vi "FindMinimumChiSquaredFastUncalibratedMethod.vi"(8 "Restrict to Positive Imaginary Part":bool=TRUE, 9 "Starting points 2":dbl[][](array[numeric])=[[1.5, 0.1], [1.5, 0.11], [1.52, 0.1]] format="%.6g", 10 "Simplex Graph":refnum<vi>, 11 "Extinction ExtinctionUncertainity Size parameter and Number ofS sizes":T1={"PAS amplitude"=[1.9915476e-09, 2.5260327e-09, 2.9463496e-09, 3.6659398e-09, 4.1150909e-09, 4.3561701e-09, 4.8158371e-09, 5.5805258e-09], "PAS amp Uncertainty"=[1.1685435e-10, 1.8562181e-10, 2.4682015e-10, 3.9807269e-10, 5.4913102e-10, 1.091901e-09, 1.2235488e-09, 1.7175431e-09], "Size parameters"=[2.4744035643168516, 2.699349342891111, 2.92429512146537, 3.149240900039629, 3.3741866786138885, 3.599132457188148, 3.8240782357624066, 4.049024014336666], "Number ofSizes"=8.0, "GeometricCrossSection"=[5.939573610693203e-10, 7.068583470577035e-10, 8.295768100885549e-10, 9.621127501618742e-10, 1.1044661672776617e-09, 1.2566370614359174e-09, 1.418625432636641e-09, 1.590431280879833e-09], "Wave Length"=349.14999, "SMPS Sizes"=[105.5, 109.4, 113.4, 117.6, 121.9, 126.3, 131.0, 135.8, 140.7, 145.9, 151.2, 156.8, 162.5, 168.5, 174.7, 181.1, 187.7, 194.6, 201.7, 209.1, 216.7, 224.7, 232.9, 241.4, 250.3, 259.5, 269.0, 278.8, 289.0, 299.6, 310.6, 322.0, 333.8, 346.0, 358.7, 371.8, 385.4, 399.5, 414.2, 429.4, 445.1, 461.4, 478.3, 495.8, 514.0, 532.8, 552.3, 572.5, 593.5, 615.3, 637.8, 661.2, 685.4, 710.5, 736.5, 763.5, 791.5], "Concentration"=array8x57[456 elements], "Double Charge Correction"=TRUE, "Extincation Factor"=1.0, "Diameter Factor"=1.0, "Diameter Offset"=0.0, "Extinction Factor Flag"=FALSE, "Diameter Factor Flag"=FALSE, "Diameter Offset Flag"=FALSE, "Sizes"=[275.0, 300.0, 325.0, 350.0, 375.0, 400.0, 425.0, 450.0], "ExtinctionOrAbsorptionOrScattering"=0, "Concentration(#/cc)"=[]} {"ExtinctionOrAbsorptionOrScattering" scale=0.0..2.0}) -> (1 "Imaginary Part from fit":dbl=0.051495699826118665, 2 "Real Part from fit":dbl=1.57799797397569, 3 "Extinction ExtinctionUncertainity Size parameter and Number ofS sizes 2":T1={"PAS amplitude"=[1.9915476e-09, 2.5260327e-09, 2.9463496e-09, 3.6659398e-09, 4.1150909e-09, 4.3561701e-09, 4.8158371e-09, 5.5805258e-09], "PAS amp Uncertainty"=[1.1685435e-10, 1.8562181e-10, 2.4682015e-10, 3.9807269e-10, 5.4913102e-10, 1.091901e-09, 1.2235488e-09, 1.7175431e-09], "Size parameters"=[2.4744035643168516, 2.699349342891111, 2.92429512146537, 3.149240900039629, 3.3741866786138885, 3.599132457188148, 3.8240782357624066, 4.049024014336666], "Number ofSizes"=8.0, "GeometricCrossSection"=[5.939573610693203e-10, 7.068583470577035e-10, 8.295768100885549e-10, 9.621127501618742e-10, 1.1044661672776617e-09, 1.2566370614359174e-09, 1.418625432636641e-09, 1.590431280879833e-09], "Wave Length"=349.14999, "SMPS Sizes"=[105.5, 109.4, 113.4, 117.6, 121.9, 126.3, 131.0, 135.8, 140.7, 145.9, 151.2, 156.8, 162.5, 168.5, 174.7, 181.1, 187.7, 194.6, 201.7, 209.1, 216.7, 224.7, 232.9, 241.4, 250.3, 259.5, 269.0, 278.8, 289.0, 299.6, 310.6, 322.0, 333.8, 346.0, 358.7, 371.8, 385.4, 399.5, 414.2, 429.4, 445.1, 461.4, 478.3, 495.8, 514.0, 532.8, 552.3, 572.5, 593.5, 615.3, 637.8, 661.2, 685.4, 710.5, 736.5, 763.5, 791.5], "Concentration"=array8x57[456 elements], "Double Charge Correction"=TRUE, "Extincation Factor"=1.0, "Diameter Factor"=1.0, "Diameter Offset"=0.0, "Extinction Factor Flag"=FALSE, "Diameter Factor Flag"=FALSE, "Diameter Offset Flag"=FALSE, "Sizes"=[275.0, 300.0, 325.0, 350.0, 375.0, 400.0, 425.0, 450.0], "ExtinctionOrAbsorptionOrScattering"=0, "Concentration(#/cc)"=[]} {"ExtinctionOrAbsorptionOrScattering" scale=0.0..2.0})   [LabVIEW 2013]
uses:
  BaesDataTypeDefinition.ctl
  RTDownhillSimplex.llb/RTDownhillSimplexGlobals.vi
panel:
  in  "Chi2 tolerance":dbl=0.001
  out "Waveform Chart":i32(graph)=60
  out "Starting points 3":dbl[][](array[numeric])=[[1.6630594557043747, 0.246532961950036], [1.4605000230939145, 0.15705446819563057], [1.5705619064033547, 0.05175990620612842]]
  in  "Downhill-Simplex parameters 2":T2={"alpha"=1.0, "beta"=0.5, "gamma"=2.0, "Maximum"=FALSE}
  out "Stopping condition flag":bool=TRUE
  out "x-y":dbl[](array[numeric])=[0.000168992022227199, 0.00018933075538369454]
  in  "buzzer":bool
  in  "Continous":bool=TRUE
  in  "sleep-time":dbl
  out "Simplex":cluster{dbl[], dbl[]}[](graph)=[{[1.57799797397569, 1.5778289819534628, 1.5778839622345557, 1.57799797397569], [0.051495699826118665, 0.05130636907073497, 0.05144020076942982, 0.051495699826118665]}]
  out "ValueInput":dbl=0.9201608571739257 format="%#_8g"
  out "ValueOutput":dbl=0.920166987183041 format="%#_8g"
  out "newSimplexPoint":dbl[](array[numeric])=[1.57799797397569, 0.051495699826118665]
  in  "Testfunction":enum16{"Rosenbrock function", "PID Controller"}(ring)=enum."PID Controller"
  in  "Downhill-Simplex parameters":T2={"alpha"=1.0, "beta"=0.5, "gamma"=2.0, "Maximum"=FALSE}
  # "Input"
  # "Output"
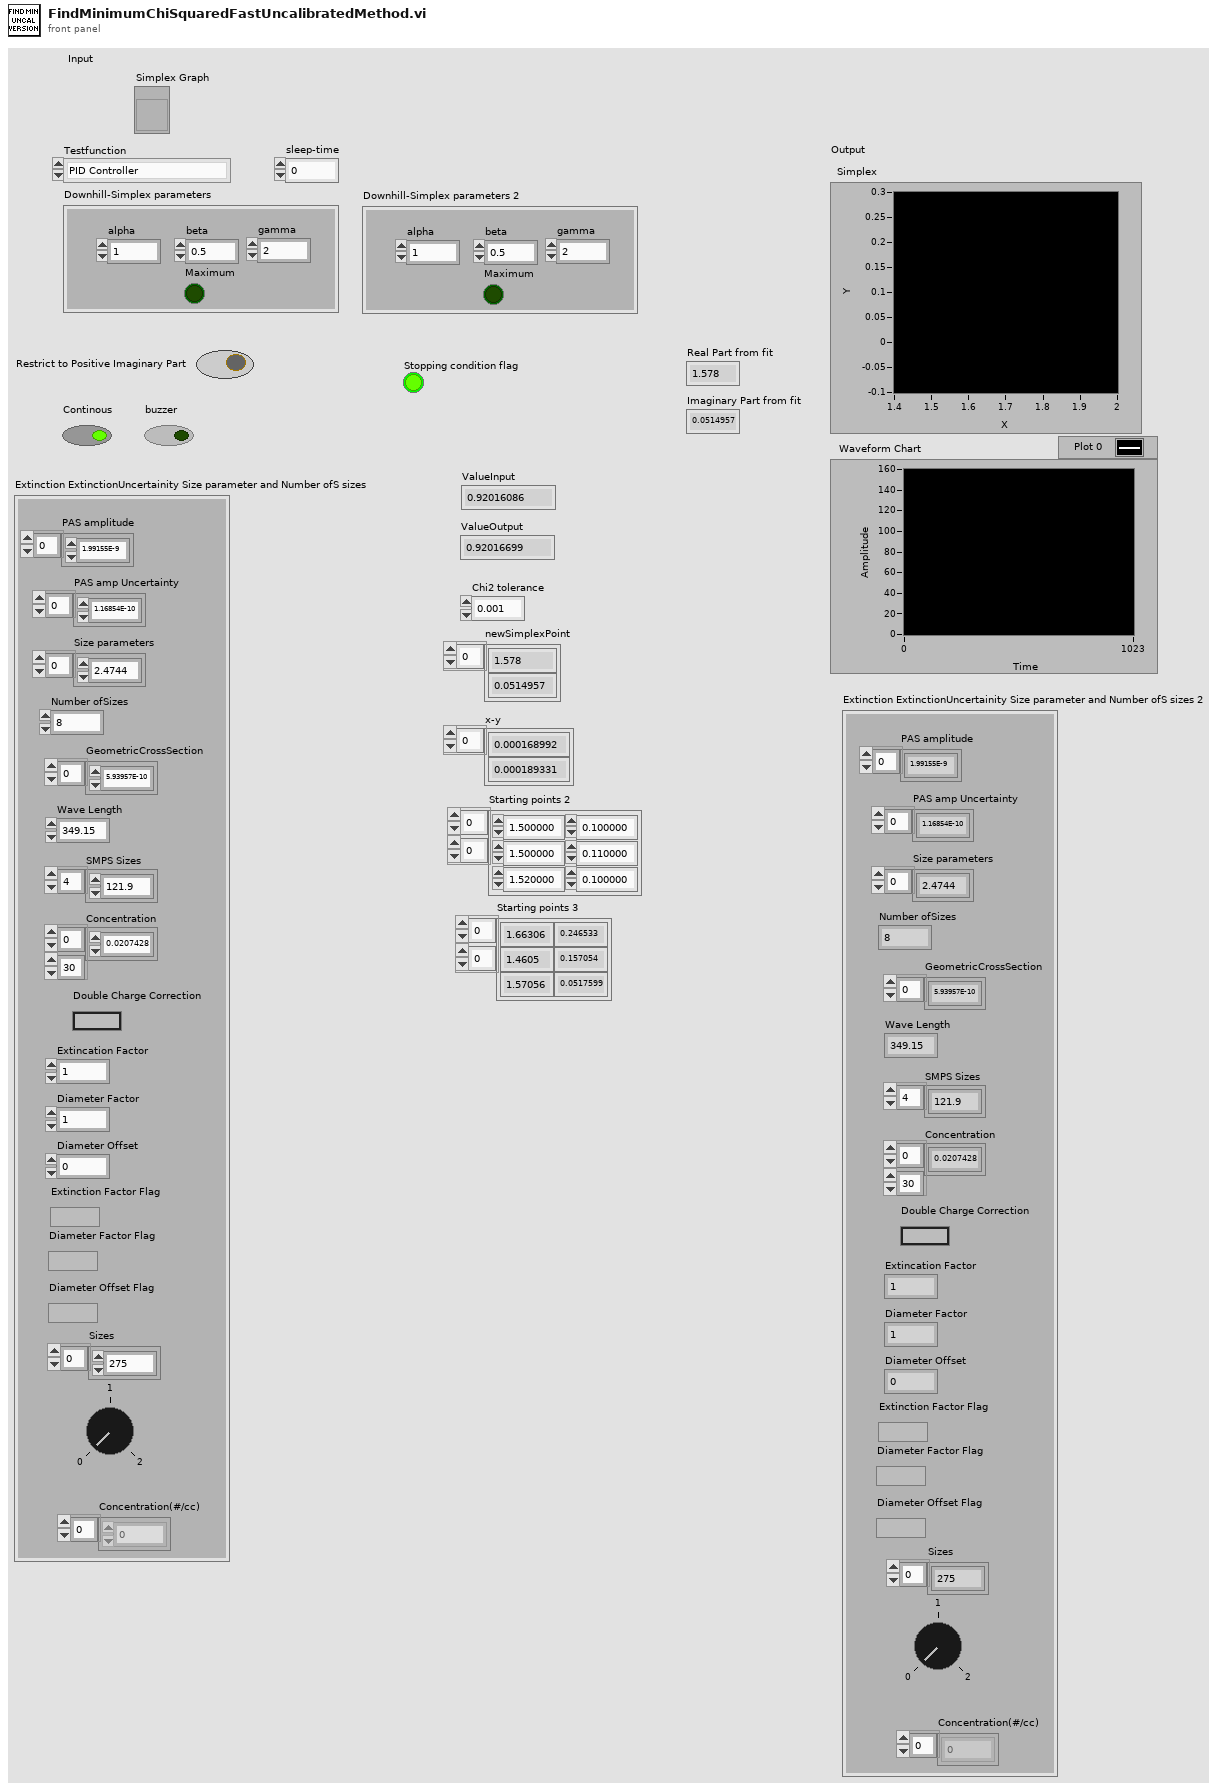
[diagram p1: front panel]
types:
  T1 = typedef "BaesDataTypeDefinition.ctl" = cluster{"PAS amplitude":dbl[], "PAS amp Uncertainty":dbl[], "Size parameters":dbl[], "Number ofSizes":dbl, "GeometricCrossSection":dbl[], "Wave Length":dbl, "SMPS Sizes":dbl[], "Concentration":dbl[][], "Double Charge Correction":bool, "Extincation Factor":dbl, "Diameter Factor":dbl, "Diameter Offset":dbl, "Extinction Factor Flag":bool, "Diameter Factor Flag":bool, "Diameter Offset Flag":bool, "Sizes":dbl[], "ExtinctionOrAbsorptionOrScattering":i8, "Concentration(#/cc)":dbl[]}
  T2 = cluster{"alpha":dbl, "beta":dbl, "gamma":dbl, "Maximum":bool}
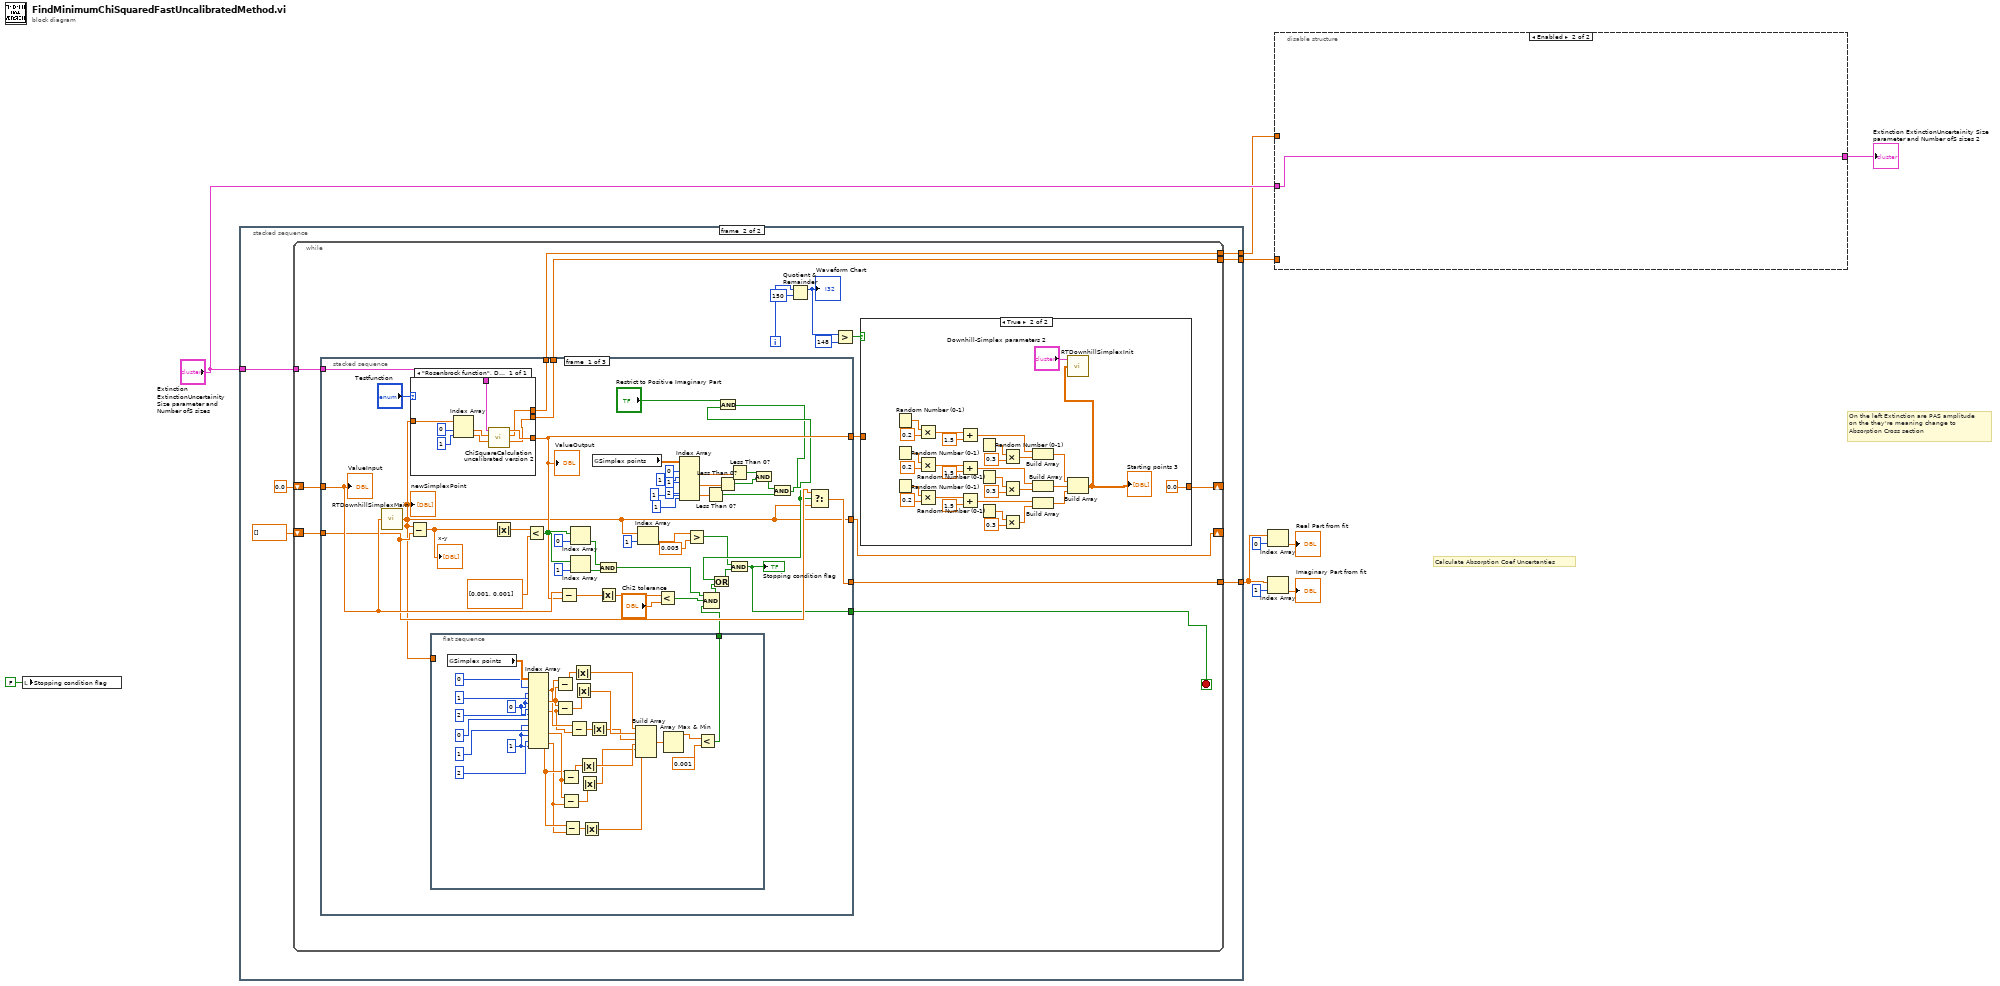
[diagram p0: block diagram]
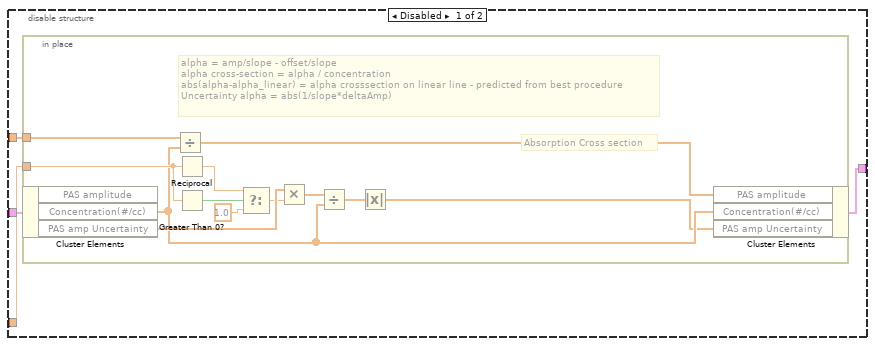
[diagram p2: hidden frame]
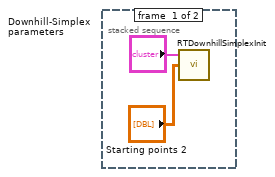
[diagram p3: hidden frame]
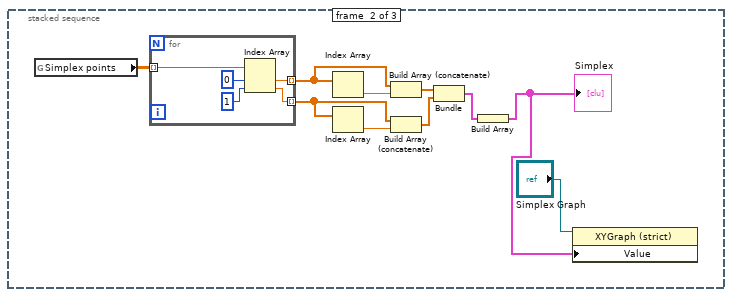
[diagram p5: hidden frame]
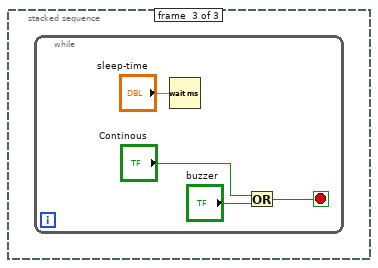
[diagram p6: hidden frame]
diagram:
  # "Calculate Absorption Coef Uncertanties"
  # "On the left Extinction are PAS amplitude\non the they're meaning change to \nAbsorption Cross section"
  n1 = local write "Stopping condition flag"(FALSE ("Stopping condition flag")) -> ()
  n2 = stacked-sequence {
    tunnel: [_ w16] -> w7
    tunnel: "Extinction ExtinctionUncertainity Size parameter and Number ofS sizes" -> [_ w15]
    tunnel: [_ w14] -> w3
    tunnel: [_ w13] -> w1
    frame #0 {
      n3 = call "RTDownhillSimplexInit.vi"("Starting points"="Starting points 2", "Downhill-Simplex parameters"="Downhill-Simplex parameters") -> ()  [unwired: 2 in]
    }
    frame #1 {
      n4 = while {
        shift-right: [w26] -> _
        shift-left: 0.0 -> [w33]
        shift-right: [w32] -> _
        shift-left: dbl[] [] ("newSimplexPoint") -> [w31]
        tunnel: [w30] -> w16
        tunnel: w15 -> [w22]
        tunnel: [w20] -> w14
        tunnel: [w19] -> w13
        i -> [w25]
        stop <- w21 stop-if-true
        n5 = stacked-sequence {
          tunnel: w33 -> [w102 _ _]
          tunnel: [w101 _ _] -> w27
          tunnel: [w71 _ _] -> w32
          tunnel: w31 -> [w85 _ _]
          tunnel: [w84 _ _] -> w30
          tunnel: w22 -> [w100 _ _]
          tunnel: [w76 _ _] -> w21
          tunnel: [w66 _ _] -> w20
          tunnel: [w65 _ _] -> w19
          frame #0 {
            n6 = call "RTDownhillSimplexMain.vi"("newSimplexValue"=w102) -> ("newSimplexPoint"=w71:dbl[])
            "newSimplexPoint" <- w71
            n7 = Subtract(x=w71, y=w85) -> (x-y=w110:dbl[])
            "x-y" <- w110
            n8 = case shown="\"Rosenbrock function\", Default" "Testfunction" {
              tunnel: w71 -> [w151]
              tunnel: [w146] -> w101
              tunnel: w100 -> [w145]
              tunnel: [w144] -> w66
              tunnel: [w143] -> w65
              frame "Rosenbrock function", Default {
                n9 = Index Array(array=w151, index #1=0 ("index"), index #2=1 ("index")) -> (element #1=w148:dbl, element #2=w147:dbl)
                n10 = call "ChiSquareCalculation uncalibrated version 2.vi"("refractive index, imaginary"=w147, "refractive index, real"=w148, "Extinction ExtinctionUncertainity Size parameter and Number ofS sizes 2"=w145) -> ("slope"=w143:dbl, "Absorption Coef Predicted Mie"=w144:dbl[], "Chi Squared"=w146:dbl)  [unwired: 5 in, 1 out]
              }
            }
            "ValueOutput" <- w101
            n11 = flat-sequence {
              tunnel: w71 -> [_]
              tunnel: [w112] -> w68
              frame #0 {
                w132 = 1 ("disabled index (col)")
                w131 = 0 ("disabled index (col)")
                n12 = global read "RTDownhillSimplexGlobals.vi" "Simplex points"() -> (w142:dbl[][])
                n13 = Index Array(array=w142, index (row) #1=0 ("index (row)"), index (col) #1=w131, index (row) #2=1 ("index (row)"), index (col) #2=w131, index (row) #3=2 ("index (row)"), index (col) #3=w131, index (row) #4=0 ("index (row)"), index (col) #4=w132, index (row) #5=1 ("index (row)"), index (col) #5=w132, index (row) #6=2 ("index (row)"), index (col) #6=w132) -> (element #1=w127:dbl, element #2=w137:dbl, element #3=w126:dbl, element #4=w124:dbl, element #5=w128:dbl, element #6=w123:dbl)
                n14 = Subtract(x=w127, y=w137) -> (x-y=w139:dbl)
                n15 = Subtract(x=w137, y=w126) -> (x-y=w136:dbl)
                n16 = Subtract(x=w124, y=w128) -> (x-y=w129:dbl)
                n17 = Subtract(x=w128, y=w123) -> (x-y=w130:dbl)
                n18 = Subtract(x=w124, y=w123) -> (x-y=w122:dbl)
                n19 = Subtract(x=w127, y=w126) -> (x-y=w125:dbl)
                n20 = Absolute Value(x=w139) -> (abs(x)=w121:dbl)
                n21 = Absolute Value(x=w136) -> (abs(x)=w120:dbl)
                n22 = Absolute Value(x=w129) -> (abs(x)=w118:dbl)
                n23 = Absolute Value(x=w130) -> (abs(x)=w117:dbl)
                n24 = Absolute Value(x=w122) -> (abs(x)=w116:dbl)
                n25 = Absolute Value(x=w125) -> (abs(x)=w119:dbl)
                n26 = Build Array(w121, w120, w119, w118, w117, w116) -> (w115:dbl[])
                n27 = Array Max & Min(array=w115) -> (max value=w114:dbl)  [unwired: 3 out]
                n28 = Less?(x=w114, y=0.001) -> (x < y?=w112:bool)
              }
            }
            n29 = Absolute Value(x=w110) -> (abs(x)=w73:dbl[])
            n30 = Less?(x=w73, y=dbl[] [0.001, 0.001]) -> (x < y?=w106:bool[])
            n31 = Subtract(x=w102, y=w101) -> (x-y=w103:dbl)
            n32 = Index Array(array=w106, index=0) -> (element=w105:bool)
            n33 = Index Array(array=w106, index=1) -> (element=w104:bool)
            n34 = global read "RTDownhillSimplexGlobals.vi" "Simplex points"() -> (w99:dbl[][])
            n35 = And(x=w105, y=w104) -> (x .and. y?=w70:bool)
            n36 = Absolute Value(x=w103) -> (abs(x)=w72:dbl)
            n37 = Index Array(array=w71, index=1) -> (element=w75:dbl)
            n38 = Less?(x=w72, y="Chi2 tolerance") -> (x < y?=w69:bool)
            n39 = Index Array(array=w99, index (row) #1=0 ("index (row)"), index (col) #1=1 ("disabled index (col)"), index (row) #2=1 ("index (row)"), index (col) #2=1 ("disabled index (col)"), index (row) #3=2 ("index (row)"), index (col) #3=1 ("disabled index (col)")) -> (element #1=w92:dbl, element #2=w91:dbl, element #3=w90:dbl)
            n40 = Greater?(x=w75, y=0.005) -> (0:w78:bool)
            n41 = Compound Arithmetic op=AND(w70, w69, w68) -> (w67:bool)
            n42 = Less Than 0?(x=w90) -> (x < 0?=w86:bool)
            n43 = Less Than 0?(x=w91) -> (x < 0?=w88:bool)
            n44 = Less Than 0?(x=w92) -> (x < 0?=w89:bool)
            n45 = And(x=w89, y=w88) -> (x .and. y?=w87:bool)
            n46 = And(x=w87, y=w86) -> (x .and. y?=w82:bool)
            n47 = And(x="Restrict to Positive Imaginary Part", y=w82) -> (x .and. y?=w81:bool)
            n48 = Or(x=w81, y=w67) -> (x .or. y?=w77:bool)
            n49 = And(x=w78, y=w77) -> (x .and. y?=w76:bool)
            "Stopping condition flag" <- w76
            n50 = Select(t=w85, s=w81, f=w71) -> (s? t:f=w84:dbl[])
            "ValueInput" <- w102
          }
          frame #1 {
            n51 = global read "RTDownhillSimplexGlobals.vi" "Simplex points"() -> (w155:dbl[][])
            n52 = for {
              tunnel: w155 -> [w166] mode=indexing
              tunnel: [w163] -> w160 mode=indexing
              tunnel: [w162] -> w157 mode=indexing
              n53 = Index Array(array=w166, index #1=0 ("index"), index #2=1 ("index")) -> (element #1=w163:dbl, element #2=w162:dbl)
            }
            n54 = Index Array(array=w160) -> (element=w161:dbl)  [unwired: 1 in]
            n55 = Index Array(array=w157) -> (element=w158:dbl)  [unwired: 1 in]
            n56 = Build Array (concatenate)(w160, w161) -> (w159:dbl[])
            n57 = Build Array (concatenate)(w157, w158) -> (w156:dbl[])
            n58 = Bundle(w159, w156) -> (w154:cluster{dbl[], dbl[]})  [unwired: 1 out]
            n59 = Build Array(w154) -> (w152:cluster{dbl[], dbl[]}[])
            "Simplex" <- w152
            n60 = property class="XYGraph (strict)"(reference="Simplex Graph", "Value"=w152) -> ()  [unwired: 1 in, 2 out]
          }
          frame #2 {
            n61 = while {
              stop <- w169 stop-if-true
              n62 = Wait (ms)(milliseconds to wait="sleep-time") -> ()  [unwired: 1 out]
              n63 = Or(x="Continous", y="buzzer") -> (x .or. y?=w169:bool)
            }
          }
        }
        n64 = Quotient & Remainder(x=w25, y=150) -> (x-y*floor(x/y)=w23:i32)  [unwired: 1 out]
        "Waveform Chart" <- w23
        n65 = Greater?(x=w23, y=148) -> (0:w28:bool)
        n66 = case shown="True" w28 {
          tunnel: [w34 0.0 ("Chi Squared")] -> w26
          tunnel: w27 -> [w34 _]
          frame False {
          }
          frame True {
            n67 = Random Number (0-1)() -> (number: 0 to 1=w53:dbl)
            n68 = Random Number (0-1)() -> (number: 0 to 1=w49:dbl)
            n69 = Random Number (0-1)() -> (number: 0 to 1=w45:dbl)
            n70 = Multiply(x=w53, y=0.2) -> (x*y=w51:dbl)
            n71 = Multiply(x=w49, y=0.2) -> (x*y=w47:dbl)
            n72 = Multiply(x=w45, y=0.2) -> (x*y=w43:dbl)
            n73 = Add(x=w51, y=1.5) -> (x+y=w41:dbl)
            n74 = Add(x=w47, y=1.5) -> (x+y=w39:dbl)
            n75 = Add(x=w43, y=1.5) -> (x+y=w37:dbl)
            n76 = Random Number (0-1)() -> (number: 0 to 1=w59:dbl)
            n77 = Random Number (0-1)() -> (number: 0 to 1=w57:dbl)
            n78 = Random Number (0-1)() -> (number: 0 to 1=w55:dbl)
            n79 = Multiply(x=w59, y=0.3) -> (x*y=w40:dbl)
            n80 = Multiply(x=w57, y=0.3) -> (x*y=w38:dbl)
            n81 = Multiply(x=w55, y=0.3) -> (x*y=w36:dbl)
            n82 = Build Array(w41, w40) -> (w62:dbl[])
            n83 = Build Array(w39, w38) -> (w61:dbl[])
            n84 = Build Array(w37, w36) -> (w60:dbl[])
            n85 = Build Array(w62, w61, w60) -> (w35:dbl[][])
            "Starting points 3" <- w35
            n86 = call "RTDownhillSimplexInit.vi"("Starting points"=w35, "Downhill-Simplex parameters"="Downhill-Simplex parameters 2") -> ()  [unwired: 2 in]
          }
        }
      }
    }
  }
  n87 = Index Array(array=w7, index=0) -> (element=→"Real Part from fit":dbl)
  n88 = Index Array(array=w7, index=1) -> (element=→"Imaginary Part from fit":dbl)
  n89 = disable-structure shown="Enabled" {
    disable-tunnel: "Extinction ExtinctionUncertainity Size parameter and Number ofS sizes" -> [w174 w187]
    disable-tunnel: w3 -> [w173 _]
    disable-tunnel: [w172 w187] -> w2
    disable-tunnel: w1 -> [w171 _]
    frame Disabled {
      n90 = in-place {
        in-place-border: w173 -> [w181]
        in-place-border: w171 -> [w184]
        # "alpha = amp/slope - offset/slope\nalpha cross-section = alpha / concentration\nabs(alpha-alpha_linear) = alpha crosssection on linear line - predicted from best procedure\nUncertainty alpha = abs(1/slope*deltaAmp)"
        # "Absorption Cross section"
        n91 = in-place-cluster #1(w174) -> ("Concentration(#/cc)"=w177:dbl[], "PAS amp Uncertainty"=w180:dbl[])  [unwired: 1 out]
        n92 = Divide(x=w181, y=w177) -> (x/y=w186:dbl[])
        n93 = Reciprocal(x=w184) -> (1/x=w183:dbl)
        n94 = Greater Than 0?(x=w184) -> (x > 0?=w185:bool)
        n95 = Select(t=w183, s=w185, f=1.0) -> (s? t:f=w179:dbl)
        n96 = Multiply(x=w180, y=w179) -> (x*y=w178:dbl[])
        n97 = Divide(x=w178, y=w177) -> (x/y=w176:dbl[])
        n98 = Absolute Value(x=w176) -> (abs(x)=w175:dbl[])
        n99 = in-place-cluster #1("PAS amplitude"=w186, "Concentration(#/cc)"=w177, "PAS amp Uncertainty"=w175) -> (w172:T1)
      }
    }
    frame Enabled {
    }
  }
  "Extinction ExtinctionUncertainity Size parameter and Number ofS sizes 2" <- w2
